vi "set current sub test.vi"(8 "error in (no error)":errorcluster, 9 "result string":string, 11 "VISA Refnum in":refnum<visa-resource-name>) -> (0 "error out":errorcluster)   [LabVIEW 2024]
uses:
  C:/Program Files/National Instruments/LabVIEW 2024/examples/Instrument IO/Serial/support/Serial - Settings.ctl
  C:/Program Files/National Instruments/LabVIEW 2024/examples/Instrument IO/Serial/support/Serial - XON-XOFF Characters.ctl
  C:/Program Files/National Instruments/LabVIEW 2024/examples/Instrument IO/Serial/support/Serial - ASCII Characters.ctl
  <vilib>/Instr/_visa.llb/VISA Configure Serial Port (Instr).vi
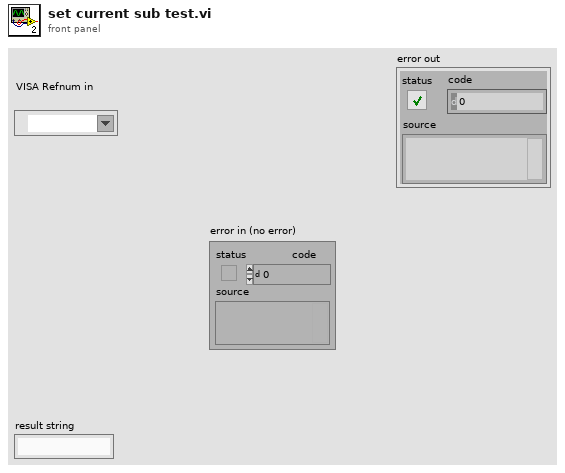
[diagram p1: front panel]
types:
  T1 = typedef "Serial - XON-XOFF Characters.ctl" = cluster{"XON":T2, "XOFF":T2}
  T2 = typedef "Serial - ASCII Characters.ctl" = enum16{"NUL", "SOH", "STX", "ETX", "EOT", "ENQ", "ACK", "BEL", "BS", "HT", "LF", "VT", "FF", "CR", "SO", "SI", "DLE", "DC1", "DC2", "DC3", "DC4", "NAK", "SYN", "ETB", "CAN", "EM", "SUB", "ESC", "FS", "GS", "RS", "US", "SP", "!", "\"", "#", "$", "%", "&", "'", "(", ")", "*", "+", ",", "- (-)", ".", "/", "0", "1", "2", "3", "4", "5", "6", "7", "8", "9", ":", ";", "<", "=", ">", "?", "@", "A", "B", "C", "D", "E", "F", "G", "H", "I", "J", "K", "L", "M", "N", "O", "P", "Q", "R", "S", "T", "U", "V", "W", "X", "Y", "Z", "[", "\\", "]", "^", "_", "`", "a", "b", "c", "d", "e", "f", "g", "h", "i", "j", "k", "l", "m", "n", "o", "p", "q", "r", "s", "t", "u", "v", "w", "x", "y", "z", "{", "|", "}", "~"}
  T3 = typedef "Serial - Settings.ctl" = cluster{"baud rate":u32, "data bits":u16, "parity":enum16{"None", "Odd", "Even", "Mark", "Space"}, "stop bits":u16, "flow control":u16}
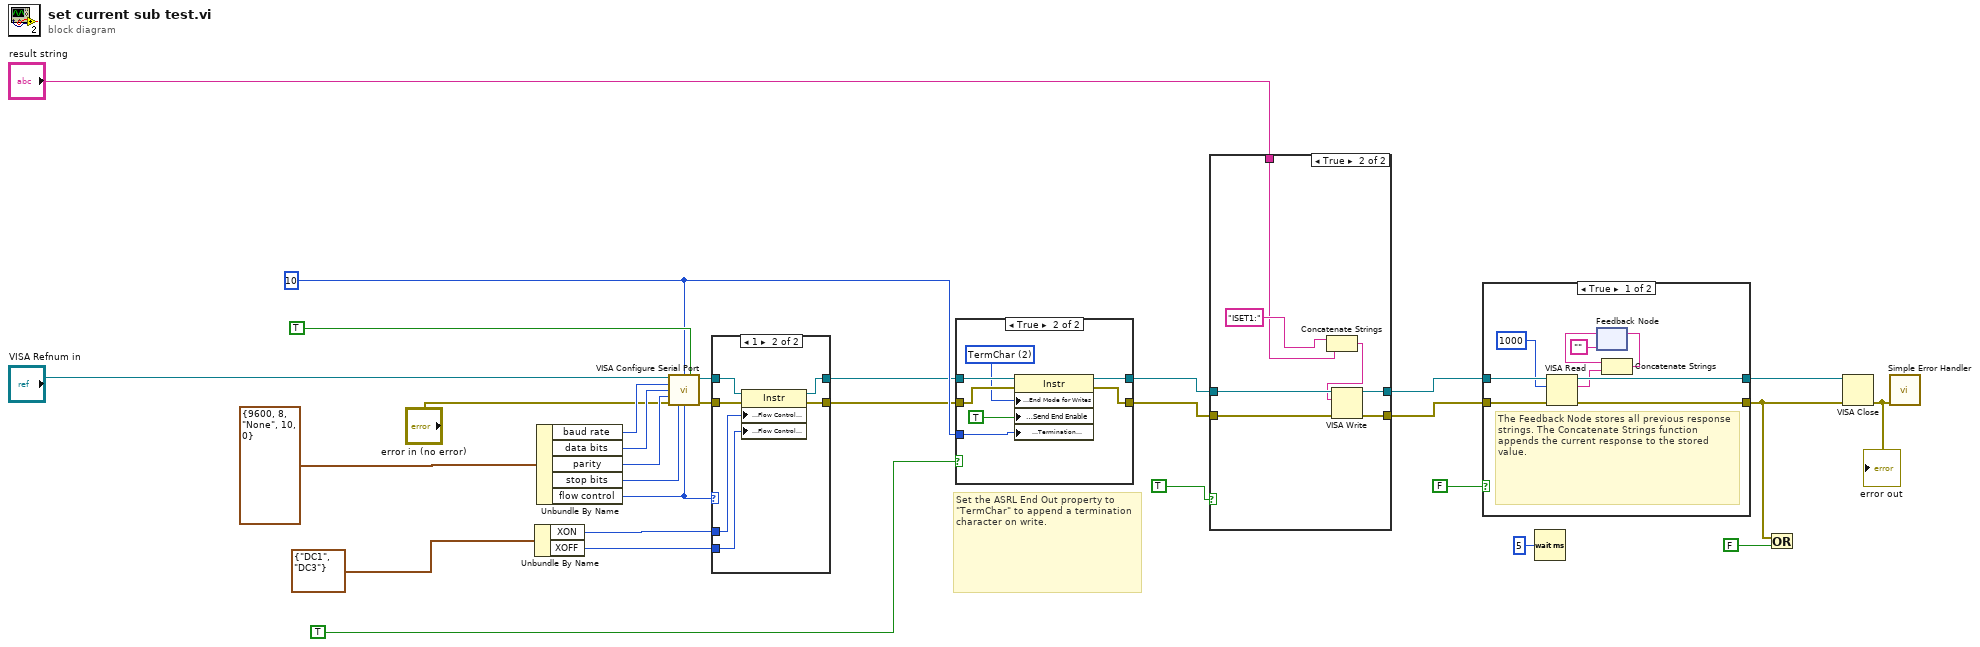
[diagram p0: block diagram]
diagram:
  w24 = u8 10 ("Termination Character")
  # "Set the ASRL End Out property to \"TermChar\" to append a termination character on write."
  n1 = Unbundle By Name(T1 {"XON"=enum."DC1", "XOFF"=enum."DC3"} ("XON/XOFF Characters 2")) -> ("XON"=w12:T2, "XOFF"=w11:T2)
  n2 = Unbundle By Name(T3 {"baud rate"=9600, "data bits"=8, "parity"=enum."None", "stop bits"=10, "flow control"=0} ("Serial Settings 2")) -> ("baud rate"=w17:u32, "data bits"=w18:u16, "parity"=w19:enum16{"None", "Odd", "Even", "Mark", "Space"}, "stop bits"=w20:u16, "flow control"=w13:u16)
  n3 = call-poly "VISA Configure Serial Port"("VISA resource name"="VISA Refnum in", "termination char\n(0xA = '\\n' = LF)"=w24, "Enable Termination\nChar (T)"=TRUE ("End Read on Termination Character?"), "baud rate (9600)"=w17, "data bits (8)"=w18, "parity (0:none)"=w19, "error in (no error)"="error in (no error)", "stop bits (10: 1 bit)"=w20, "flow control (0:none)"=w13) -> ("VISA resource name out"=w21:refnum<visa-resource-name>, "error out"=w22:errorcluster)  [unwired: 1 in, 4 out]
  n4 = case shown="1" w13 {
    tunnel: [w31 w38] -> w10
    tunnel: [w32 w37] -> w8
    tunnel: w22 -> [w31 w36]
    tunnel: w21 -> [w32 w35]
    tunnel: w12 -> [_ w34]
    tunnel: w11 -> [_ w33]
    frame Default {
    }
    frame 1 {
      n5 = property class="Instr"(reference=w35, error in=w36, "Serial Settings:Flow Control XON Character"=w34, "Serial Settings:Flow Control XOFF Character"=w33) -> (reference out=w37:refnum<visa-resource-name>, error out=w38:errorcluster)
    }
  }
  n6 = case shown="True" TRUE ("End Write on Termination Character?") {
    tunnel: w8 -> [w39 w47]
    tunnel: w10 -> [w40 w46]
    tunnel: [w39 w45] -> w7
    tunnel: [w40 w44] -> w9
    tunnel: w24 -> [_ w42]
    frame False {
    }
    frame True {
      w43 = u16 2 items=["None", "LastBit", "TermChar", "Break"] ("Serial Settings:Serial End Mode for Writes")
      n7 = property class="Instr"(reference=w47, error in=w46, "Serial Settings:End Mode for Writes"=w43, "Message Based Settings:Send End Enable"=TRUE, "Message Based Settings:Termination Character"=w42) -> (reference out=w45:refnum<visa-resource-name>, error out=w44:errorcluster)
    }
  }
  n8 = case shown="True" TRUE ("Write 2") {
    tunnel: w7 -> [w49 w56]
    tunnel: w9 -> [w48 w55]
    tunnel: [w49 w54] -> w6
    tunnel: [w48 w53] -> w5
    tunnel: "result string" -> [_ w50]
    frame False {
    }
    frame True {
      n9 = Concatenate Strings("ISET1:" ("string"), w50) -> (w51:string)
      n10 = VISA Write(VISA resource name=w56, write buffer=w51, error in (no error)=w55) -> (VISA resource name out=w54:refnum<visa-resource-name>, error out=w53:errorcluster)  [unwired: 1 out]
    }
  }
  n11 = case shown="True" FALSE ("Read in") {
    tunnel: [w63 w67] -> w14
    tunnel: w6 -> [w65 w67]
    tunnel: [w61 w66] -> w15
    tunnel: w5 -> [w64 w66]
    frame True {
      # "The Feedback Node stores all previous response strings. The Concatenate Strings function appends the current response to the stored value."
      n12 = VISA Read(VISA resource name=w65, byte count=u32 1000 ("Read Count"), error in (no error)=w64) -> (VISA resource name out=w63:refnum<visa-resource-name>, read buffer=w60:string, error out=w61:errorcluster)  [unwired: 1 out]
      n13 = feedback #1("") -> (w59:string)
      n14 = Concatenate Strings(w59, w60) -> (w58:string)
      n15 = feedback-in #1(w58) -> ()
    }
    frame False {
    }
  }
  n16 = Wait (ms)(milliseconds to wait=u32 5) -> ()  [unwired: 1 out]
  n17 = Or(x=w15, y=FALSE ("Stop")) -> ()  [unwired: 1 out]
  n18 = VISA Close(VISA resource name=w14, error in (no error)=w15) -> (error out=w2:errorcluster)
  "error out" <- w2
  n19 = call <vilib>:"Simple Error Handler.vi"("error in (no error)"=w2) -> ()  [unwired: 1 in, 8 out]
